vi "New Data Item.vi"(8 "error in (no error)":errorcluster, 10 "Item ID":string, 11 "node in":refnum<k20>) -> (0 "error out":errorcluster, 3 "Data Item":refnum<class "Data Item.lvclass">)   [LabVIEW 2026, in "VILab.lvlib"]
uses:
  VILab.lvlib
  Classes/Data Item/Data Item.lvclass
  Classes/Element/Element.lvclass
  <resource>/objmgr/DOMUserDefRef.rc
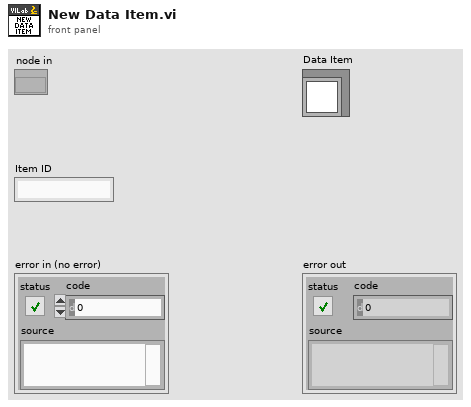
[diagram p1: front panel]
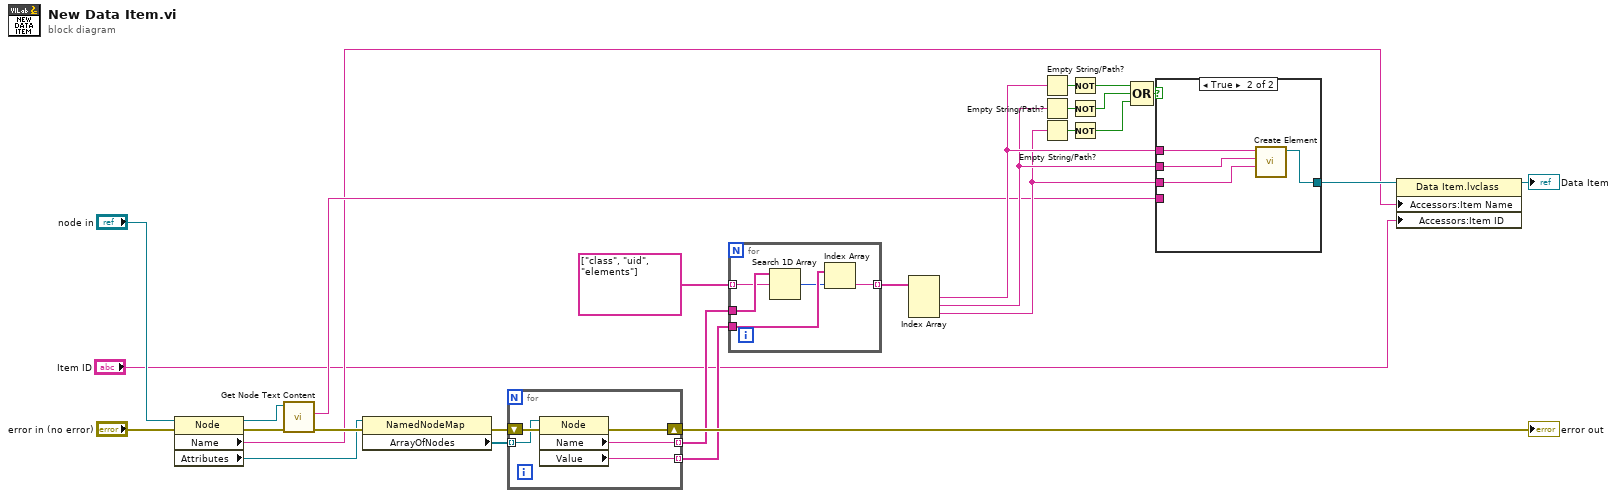
[diagram p0: block diagram]
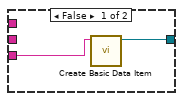
[diagram p2: hidden frame]
diagram:
  n1 = property class="Node"(reference="node in", error in="error in (no error)") -> (reference out=w16:refnum<k20>, error out=w25:errorcluster, "Name"=w3:string, "Attributes"=w17:refnum<k20>)
  n2 = call "Get Node Text Content.vi"("error in (no error)"=w25, "node in"=w16) -> ("error out"=w24:errorcluster, "node text"=w4:string)  [unwired: 7 in, 1 out]
  n3 = property class="NamedNodeMap"(reference=w17, error in=w24) -> (error out=w28:errorcluster, "ArrayOfNodes"=w23:refnum<k20>[])  [unwired: 1 out]
  n4 = for {
    tunnel: w23 -> [w32] mode=indexing
    tunnel: [w31] -> w22 mode=indexing
    tunnel: [w30] -> w21 mode=indexing
    shift-right: [w29] -> w26
    shift-left: w28 -> [w33]
    n5 = property class="Node"(reference=w32, error in=w33) -> (error out=w29:errorcluster, "Name"=w31:string, "Value"=w30:string)  [unwired: 1 out]
  }
  "error out" <- w26
  n6 = for {
    tunnel: w22 -> [w38]
    tunnel: w21 -> [w36]
    tunnel: string[] ["class", "uid", "elements"] -> [w37] mode=indexing
    tunnel: [w34] -> w19 mode=indexing
    n7 = Search 1D Array(1D array=w38, element=w37) -> (index of element=w35:i32)  [unwired: 1 in]
    n8 = Index Array(array=w36, index=w35) -> (element=w34:string)
  }
  n9 = Index Array(array=w19) -> (element #1=w7:string, element #2=w6:string, element #3=w5:string)  [unwired: 3 in]
  n10 = Empty String/Path?(string/path=w7) -> (empty?=w15:bool)
  n11 = Empty String/Path?(string/path=w6) -> (empty?=w14:bool)
  n12 = Empty String/Path?(string/path=w5) -> (empty?=w10:bool)
  n13 = Not(x=w15) -> (.not. x?=w13:bool)
  n14 = Not(x=w14) -> (.not. x?=w12:bool)
  n15 = Not(x=w10) -> (.not. x?=w9:bool)
  n16 = Compound Arithmetic op=OR(w13, w12, w9) -> (w11:bool)
  n17 = case shown="True" w11 {
    tunnel: w6 -> [_ w44]
    tunnel: [w40 w43] -> w8
    tunnel: w4 -> [w39 _]
    tunnel: w7 -> [_ w42]
    tunnel: w5 -> [_ w41]
    frame False {
      n18 = call "Create Basic Data Item.vi"("Content"=w39) -> ("New Data Item"=w40:refnum<class "Data Item.lvclass">)  [unwired: 10 in]
    }
    frame True {
      n19 = call "Create Element.vi"("elements"=w41, "uid"=w44, "class"=w42) -> ("Element"=w43:refnum<class "Element.lvclass">)  [unwired: 8 in]
    }
  }
  n20 = property class="Data Item.lvclass"(reference=w8, "Accessors:Item Name"=w3, "Accessors:Item ID"="Item ID") -> (reference out=→"Data Item":refnum<class "Data Item.lvclass">)  [unwired: 1 in, 1 out]
